vi "Andrew_Struthers_ThermistorLab.vi"() -> ()   [LabVIEW 2018]
uses:
  <vilib>/express/express shared/transition.llb/Dynamic To Waveform Array.vi
  <vilib>/express/express arith-compare/Formula/Block/exnFormulaBlock how many pts in the wave.vi
  <vilib>/express/express shared/ex_Modify Signal Name.vi
  <vilib>/express/express shared/transition.llb/Waveform Array To Dynamic.vi
  <vilib>/express/express arith-compare/Formula/XNode/ExpressFormulaBlockNode.xnode
panel:
  in  "?":bool
  out "Temperature":dbl
  out "Gauge":dbl(knob) scale=60.0..200.0
  out "Volts":dbl
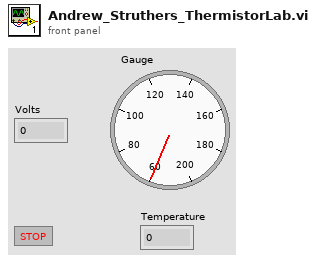
[diagram p1: front panel]
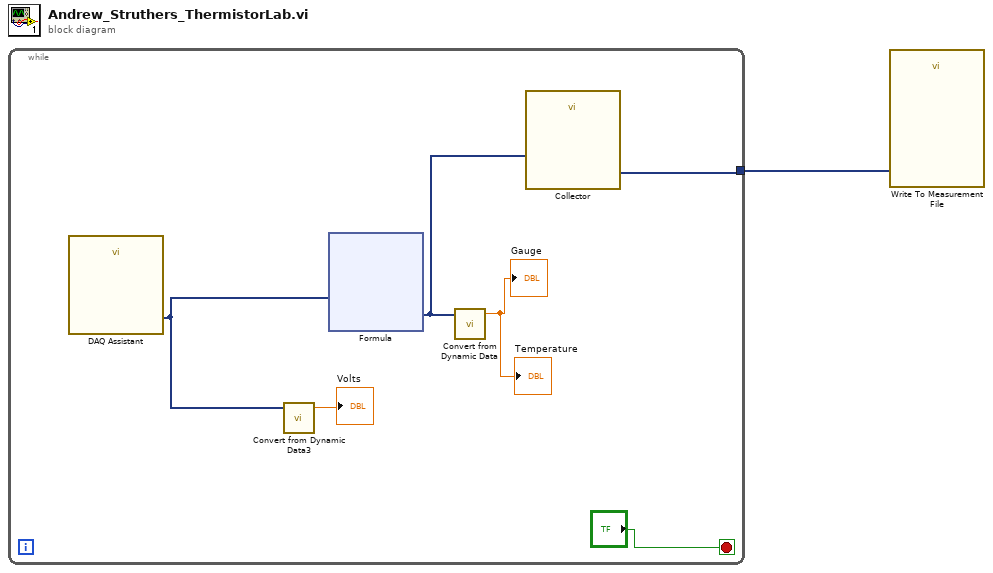
[diagram p0: block diagram]
diagram:
  n1 = while {
    tunnel: [w4] -> w1
    stop <- "?" stop-if-true
    n2 = call "DAQ Assistant"() -> ("data"=w2:dynamicdata)  [unwired: 17 in, 2 out]
    n3 = call "Convert from Dynamic Data3"("Dynamic Data Type"=w2) -> ("Scalar"=→"Volts":dbl)  [unwired: 3 in]
    n4 = xnode "Formula"("V"=w2) -> ("Result"=w7:dynamicdata)  [unwired: 1 in, 1 out]
    n5 = call "Convert from Dynamic Data"("Dynamic Data Type"=w7) -> ("Scalar"=→"Gauge" →"Temperature":dbl)  [unwired: 3 in]
    n6 = call "Collector"("Signals"=w7) -> ("Collected Signals"=w4:dynamicdata)  [unwired: 9 in, 1 out]
  }
  n7 = call "Write To Measurement File"("Signals"=w1) -> ()  [unwired: 16 in, 3 out]
